vi "Base64 Decode.vi"(1 "base64 string":string) -> (0 "normal string":string)   [LabVIEW 2015, in "Car Wash.lvlib" / "Tools_String.lvlib"]
doc: "Decodes a Base64-encoded string"
uses:
  Tools_String.lvlib
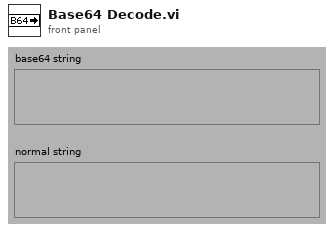
[diagram p1: front panel]
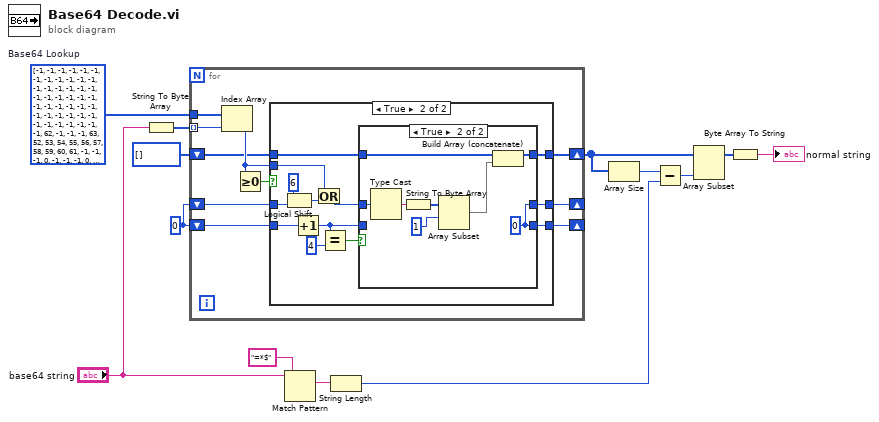
[diagram p0: block diagram]
diagram:
  w11 = 0
  w12 = i8[] [-1, -1, -1, -1, -1, -1, -1, -1, -1, -1, -1, -1, -1, -1, -1, -1, -1, -1, -1, -1, -1, -1, -1, -1, -1, -1, -1, -1, -1, -1, -1, -1, -1, -1, -1, -1, -1, -1, -1, -1, -1, -1, -1, 62, -1, -1, -1, 63, 52, 53, 54, 55, 56, 57, 58, 59, 60, 61, -1, -1, -1, 0, -1, -1, -1, 0, 1, 2, 3, 4, 5, 6, 7, 8, 9, 10, 11, 12, 13, 14, 15, 16, 17, 18, 19, 20, 21, 22, 23, 24, 25, -1, -1, -1, -1, -1, -1, 26, 27, 28, 29, 30, 31, 32, 33, 34, 35, 36, 37, 38, 39, 40, 41, 42, 43, 44, 45, 46, 47, 48, 49, 50, 51, -1, -1, -1, -1, -1, -1, -1, -1, -1, -1, -1, -1, -1, -1, -1, -1, -1, -1, -1, -1, -1, -1, -1, -1, -1, -1, -1, -1, -1, -1, -1, -1, -1, -1, -1, -1, -1, -1, -1, -1, -1, -1, -1, -1, -1, -1, -1, -1, -1, -1, -1, -1, -1, -1, -1, -1, -1, -1, -1, -1, -1, -1, -1, -1, -1, -1, -1, -1, -1, -1, -1, -1, -1, -1, -1, -1, -1, -1, -1, -1, -1, -1, -1, -1, -1, -1, -1, -1, -1, -1, -1, -1, -1, -1, -1, -1, -1, -1, -1, -1, -1, -1, -1, -1, -1, -1, -1, -1, -1, -1, -1, -1, -1, -1, -1, -1, -1, -1, -1, -1, -1, -1, -1, -1, -1, -1, -1, -1, -1, -1, -1, -1, -1]  # Base64 Lookup
  n1 = String To Byte Array(string="base64 string") -> (unsigned byte array=w13:u8[])
  n2 = for {
    tunnel: w13 -> [w23] mode=indexing
    tunnel: w12 -> [w22]
    shift-right: [w16] -> _
    shift-left: w11 -> [w17]
    shift-right: [w21] -> _
    shift-left: w11 -> [w20]
    shift-right: [w14] -> w5
    shift-left: u8[] [] -> [w15]
    n3 = Index Array(array=w22, index=w23) -> (element=w19:i8)
    n4 = Greater Or Equal To 0?(x=w19) -> (x >= 0?=w18:bool)
    n5 = case shown="True" w18 {
      tunnel: w19 -> [_ w39]
      tunnel: w20 -> [w25 w38]
      tunnel: [w25 w32] -> w21
      tunnel: w17 -> [w24 w35]
      tunnel: [w24 w29] -> w16
      tunnel: w15 -> [w26 w28]
      tunnel: [w26 w27] -> w14
      frame False {
      }
      frame True {
        n6 = Logical Shift(y=i16 6, x=w38) -> (x << y=w37:i32)
        n7 = Increment(x=w35) -> (x+1=w30:i32)
        n8 = Or(x=w39, y=w37) -> (x .or. y?=w31:i32)
        n9 = Equal?(x=w30, y=4) -> (x = y?=w33:bool)
        n10 = case shown="True" w33 {
          tunnel: [w42 w50] -> w32
          tunnel: w31 -> [w42 w49]
          tunnel: w30 -> [w41 _]
          tunnel: [w41 w50] -> w29
          tunnel: w28 -> [w40 w45]
          tunnel: [w40 w43] -> w27
          frame False {
          }
          frame True {
            w50 = 0
            n11 = Type Cast(x=w49) -> (*(type *) &x=w48:string)  [unwired: 1 out]
            n12 = String To Byte Array(string=w48) -> (unsigned byte array=w47:u8[])
            n13 = Array Subset(array=w47, index=1) -> (w44:u8[])  [unwired: 1 in]
            n14 = Build Array (concatenate)(w45, w44) -> (w43:u8[])
          }
        }
      }
    }
  }
  n15 = Match Pattern(string="base64 string", regular expression="=*$") -> (match substring=w7:string)  [unwired: 4 out]
  n16 = String Length(string=w7) -> (length=w3:i32)
  n17 = Array Size(array=w5) -> (size(s)=w4:i32)
  n18 = Subtract(x=w4, y=w3) -> (x-y=w2:i32)
  n19 = Array Subset(array=w5, length=w2) -> (w6:u8[])  [unwired: 1 in]
  n20 = Byte Array To String(unsigned byte array=w6) -> (string=→"normal string":string)
